vi "Vision Processing.vi"(4 "error in":errorcluster, 7 "Image Size":T6=enum."320x240") -> ()   [LabVIEW 2015]
doc: "This VI runs in parallel to other tasks. It gets images from the camera, processes them for color or shape and use that information to affect robot behavior."
uses:
  <vilib>/Rock Robotics/WPI/Camera/WPI_CameraImageSize.ctl
  Program Files (x86)/National Instruments/LabVIEW 2015/examples/FRC/roboRIO/Vision/2016 Vision Example/Vision Support Code/Camera Types.ctl
  <vilib>/Rock Robotics/WPI/Camera/WPI_CameraFrameRate.ctl
  Robot Global Data.vi
  <vilib>/vision/NI_Vision_Development_Module.lvlib
panel:
  out "Targets Angles":dbl[](array[numeric])
  in  "LED Color":T1={"Hue"={23.67058792990901, 48.923317529462665}, "Sat"={66.78571428571429, 255.0}, "Val"={48.571428571428584, 255.0}} {"Hue" scale=0.0..255.0 scale format="%#_3g"}
  out "Qualified Particles":i32
  in  "Score Threshold":dbl=75.0
  in  "Aspect Fudge Factor":dbl=1.0
  in  "Min Score Threshold":i32=75
  in  "Camera Type":T2=enum."MS HD3000 square"
  in  "Emphasize Limit Tests":bool=TRUE
  out "Masked":T3(plugin-control)
  out "Original Image":T3(plugin-control)
  in  "Display Images":bool
  out "Sorted Particle Scores":T4(array[cluster]) {"Moment Factor" format="%#_3g"; "Aspect Ratio" format="%#_3g"; "Area to CH" format="%#_3g"; "X" format="%#_3g"; "Y" format="%#_3g"}
  out "Highest Avg Score":dbl
  out "Detected Targets":T5(array[cluster]) {"Normalized Rect"."Numeric 5" format="%#_2g"; "Normalized Rect"."Numeric 3" format="%#_2g"; "Normalized Rect"."Numeric 2" format="%#_2g"; "Normalized Rect"."Numeric" format="%#_2g"}
  # "Density Profile"
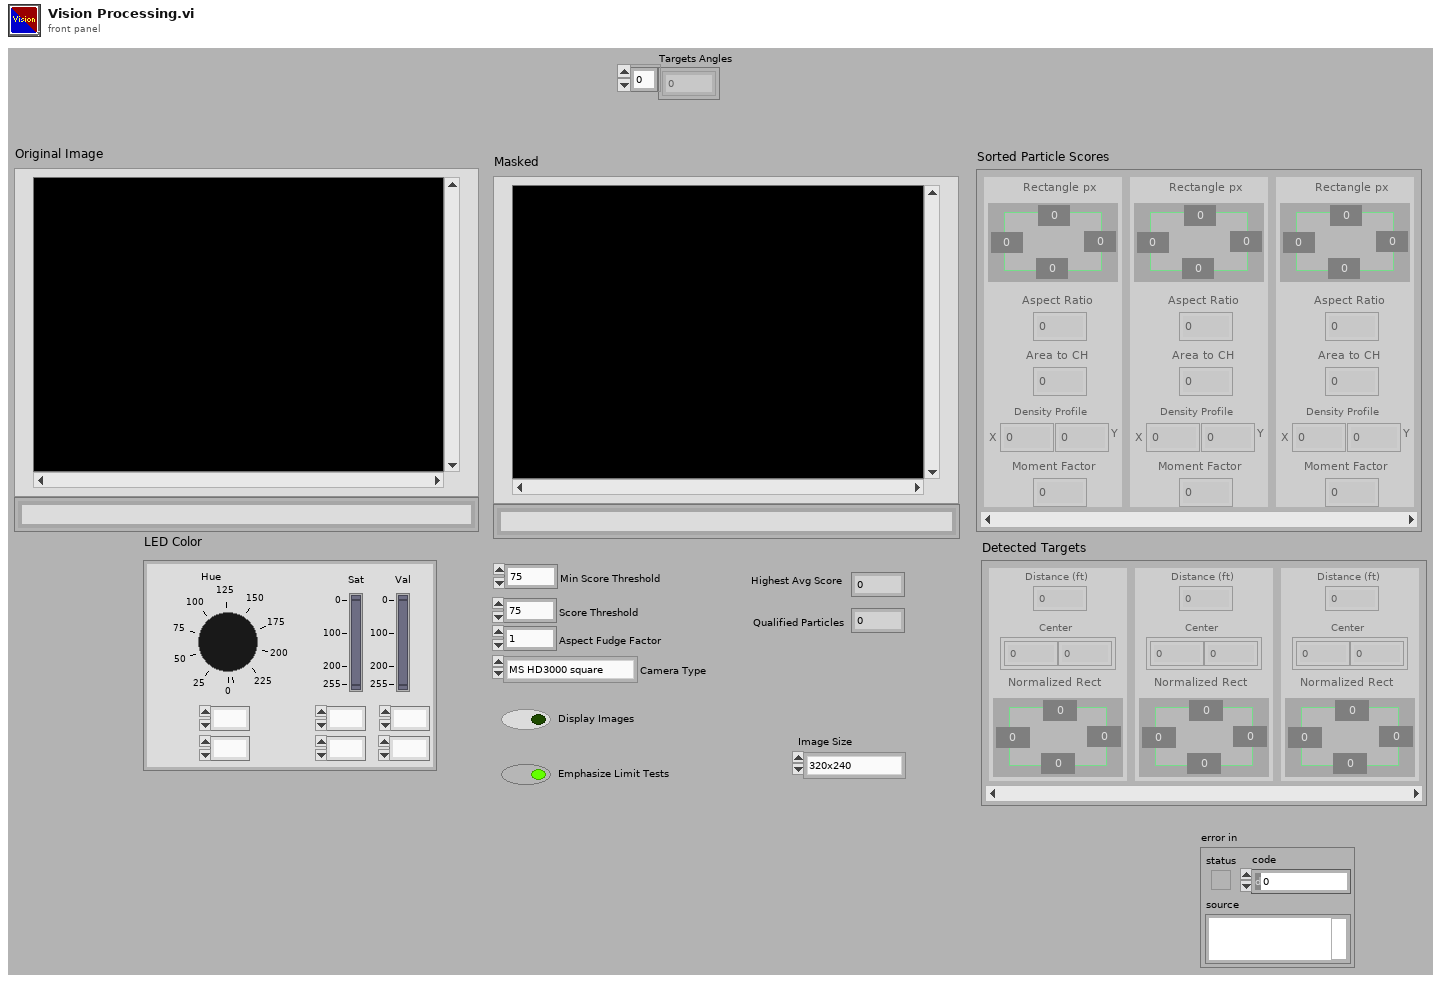
[diagram p1: front panel]
types:
  T1 = cluster{"Hue":cluster{dbl, dbl}, "Sat":cluster{dbl, dbl}, "Val":cluster{dbl, dbl}}
  T2 = typedef "Camera Types.ctl" = enum16{"206", "1011", "1013", "MS HD3000 square", "MS HD3000 640x480"}
  T3 = typedef "IMAQ Image.ctl" = refnum<image>
  T4 = cluster{"Rectangle px":cluster{"Numeric":dbl, "Numeric 2":dbl, "Numeric 3":dbl, "Numeric 5":dbl}, "Aspect Ratio":dbl, "Area to CH":dbl, "X":dbl, "Y":dbl, "Moment Factor":dbl}[]
  T5 = cluster{"Distance (ft)":dbl, "Center":cluster{dbl, dbl}, "Normalized Rect":cluster{"Numeric":dbl, "Numeric 2":dbl, "Numeric 3":dbl, "Numeric 5":dbl}}[]
  T6 = typedef "WPI_CameraImageSize.ctl" = enum16{"640x480", "320x240", "160x120", "Custom"}
  T7 = typedef "Particle Parameters" = i32
  T8 = typedef "Image Type" = u32
  T9 = typedef "WPI_CameraFrameRate.ctl" = u32
  T10 = typedef "WPI_CameraDevRef.ctl" = cluster{"Camera Address":string, "CameraStatus":errorcluster}
  T11 = cluster{"Bounding box":cluster{"left":dbl, "top":dbl, "right":dbl, "bottom":dbl}, "Aspect Ratio":dbl, "Area to CH":dbl, "X Mask":dbl, "Y Mask":dbl, "Moment":dbl}[]
  T12 = cluster{"Rectangle":cluster{"Numeric":dbl, "Numeric 2":dbl, "Numeric 3":dbl, "Numeric 5":dbl}, "L":dbl, "Area to CH":dbl, "X":dbl, "Y":dbl, "Moment Factor":dbl}[]
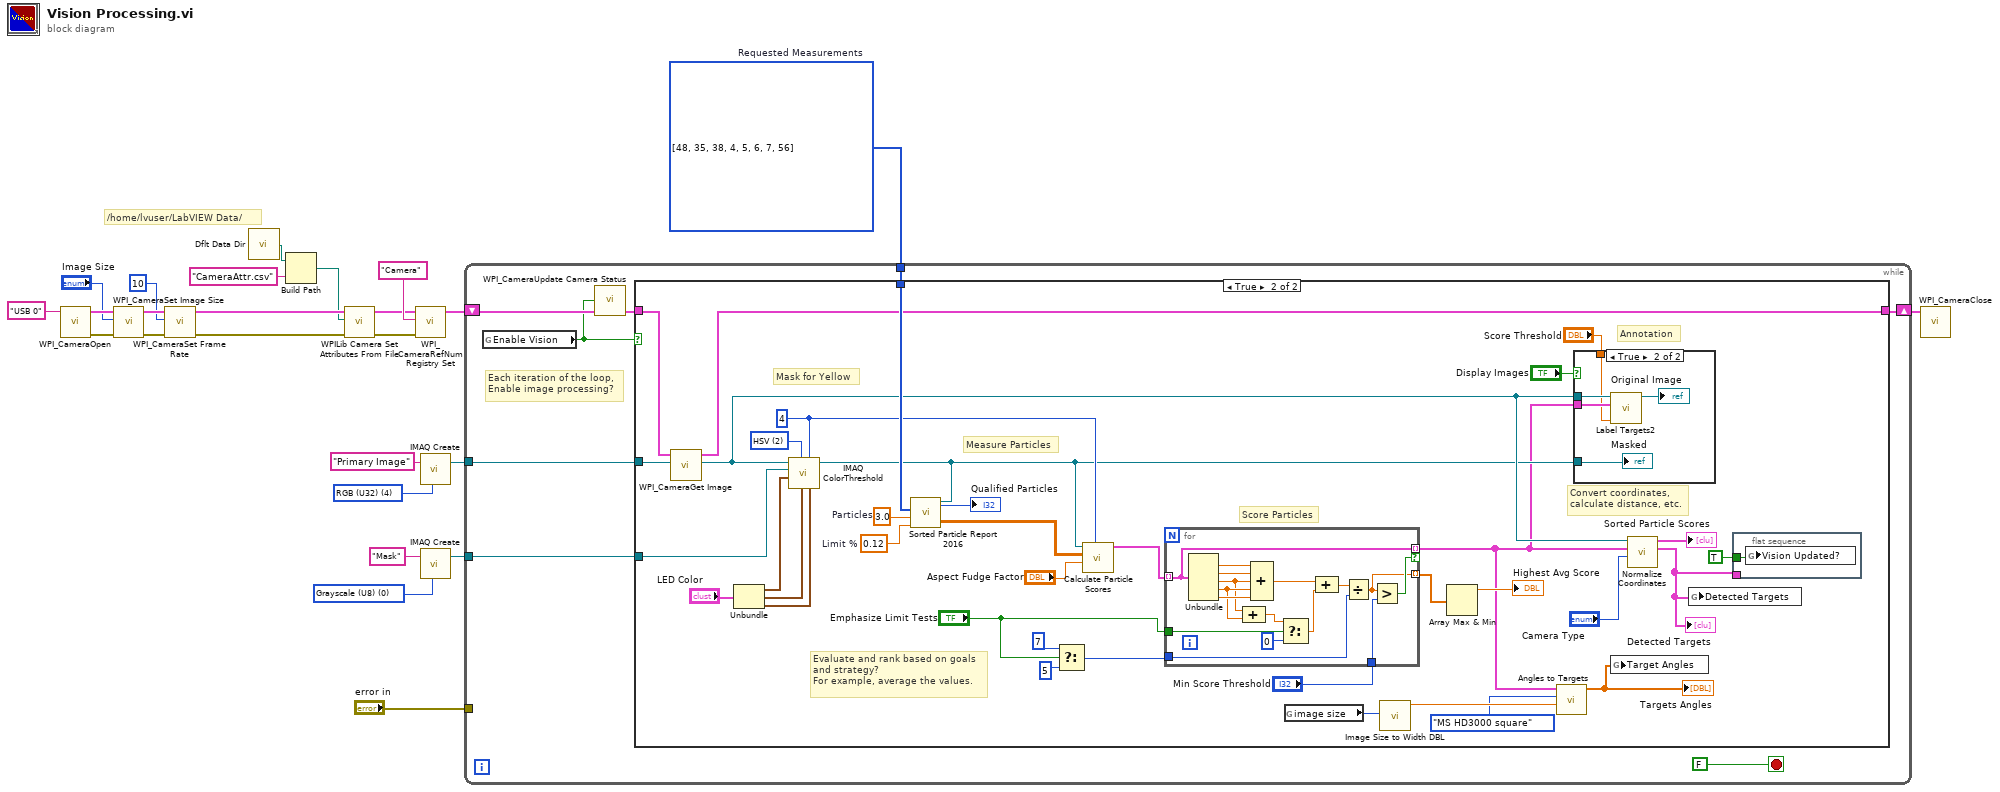
[diagram p0: block diagram]
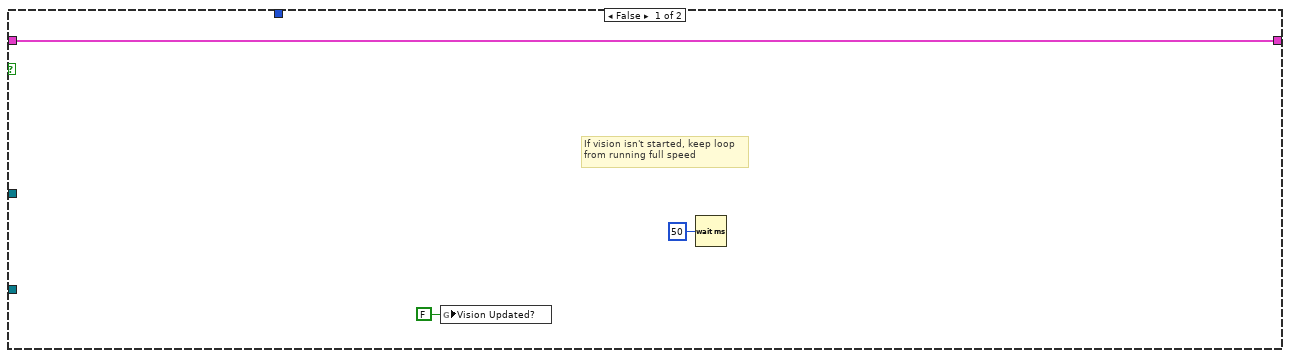
[diagram p2: hidden frame]
diagram:
  w1 = T7[] [48, 35, 38, 4, 5, 6, 7, 56] items=["Center of Mass X", "Center of Mass Y", "First Pixel X", "First Pixel Y", "Bounding Rect Left", "Bounding Rect Top", "Bounding Rect Right", "Bounding Rect Bottom", "Max Feret Diameter Start X", "Max Feret Diameter Start Y", "Max Feret Diameter End X", "Max Feret Diameter End Y", "Max Horiz. Segment Length Left", "Max Horiz. Segment Length Right", "Max Horiz. Segment Length Row", "-", "Bounding Rect Width", "Bounding Rect Height", "Bounding Rect Diagonal", "Perimeter", "Convex Hull Perimeter", "Holes' Perimeter", "Max Feret Diameter", "Equivalent Ellipse Major Axis", "Equivalent Ellipse Minor Axis", "Equivalent Ellipse Minor Axis (Feret)", "Equivalent Rect Long Side", "Equivalent Rect Short Side", "Equivalent Rect Diagonal", "Equivalent Rect Short Side (Feret)", "Average Horiz. Segment Length", "Average Vert. Segment Length", "Hydraulic Radius", "Waddel Disk Diameter", "-", "Area", "Holes' Area", "Particle & Holes' Area", "Convex Hull Area", "Image Area", "-", "Number of Holes", "Number of Horiz. Segments", "Number of Vert. Segments", "-", "Orientation", "Max Feret Diameter Orientation", "-", "% Area/Image Area", "% Area/(Particle & Holes' Area)", "Ratio of Equivalent Ellipse Axes", "Ratio of Equivalent Rect Sides", "-", "Elongation Factor", "Compactness Factor", "Heywood Circularity Factor", "Type Factor", "-", "Sum X", "Sum Y", "Sum XX", "Sum XY", "Sum YY", "Sum XXX", "Sum XXY", "Sum XYY", "Sum YYY", "-", "Moment of Inertia XX", "Moment of Inertia XY", "Moment of Inertia YY", "Moment of Inertia XXX", "Moment of Inertia XXY", "Moment of Inertia XYY", "Moment of Inertia YYY", "Norm. Moment of Inertia XX", "Norm. Moment of Inertia XY", "Norm. Moment of Inertia YY", "Norm. Moment of Inertia XXX", "Norm. Moment of Inertia XXY", "Norm. Moment of Inertia XYY", "Norm. Moment of Inertia YYY", "Hu Moment 1", "Hu Moment 2", "Hu Moment 3", "Hu Moment 4", "Hu Moment 5", "Hu Moment 6", "Hu Moment 7"]  # Requested Measurements
  w4 = T8 0 items=["Grayscale (U8)", "Grayscale (I16)", "Grayscale (SGL)", "Complex (CSG)", "RGB (U32)", "HSL (U32)", "RGB (U64)", "Grayscale (U16)"] ("Image Type")
  w25 = T8 4 items=["Grayscale (U8)", "Grayscale (I16)", "Grayscale (SGL)", "Complex (CSG)", "RGB (U32)", "HSL (U32)", "RGB (U64)"] ("Image Type")
  # "/home/lvuser/LabVIEW Data/"
  n1 = call <vilib>:"WPI_CameraOpen.vi"("Camera Address"="USB 0" ("format string")) -> ("error out"=w19:errorcluster, "CameraDevRef"=w20:T10)  [unwired: 1 in, 8 out]
  n2 = call <vilib>:"WPI_CameraSet Image Size.vi"("error in (no error)"=w19, "Image Size"="Image Size", "CameraDevRef"=w20) -> ("error out"=w18:errorcluster, "CameraDevRef Out"=w21:T10)  [unwired: 1 in, 6 out]
  n3 = call <vilib>:"WPI_CameraSet Frame Rate.vi"("error in (no error)"=w18, "Frame Rate (fps)"=T9 10, "CameraDevRef"=w21) -> ("error out"=w11:errorcluster, "CameraDevRef Out"=w12:T10)  [unwired: 7 out]
  n4 = call <vilib>:"Dflt Data Dir.vi"() -> ("App:Default Data Directory"=w8:path)
  n5 = Build Path(base path=w8, name or relative path="CameraAttr.csv") -> (appended path=w7:path)
  n6 = call "WPILib Camera Set Attributes From File.vi"("error in"=w11, "Config Path"=w7, "CameraDevRef"=w12) -> ("error out"=w9:errorcluster, "CameraDevRef"=w10:T10)  [unwired: 7 in]
  n7 = call <vilib>:"WPI_CameraRefNum Registry Set.vi"("error in (no error)"=w9, "refnum name"="Camera", "CameraDevRef"=w10) -> ("CameraDevRef"=w16:T10)  [unwired: 1 in, 7 out]
  n8 = call "IMAQ Create"("Image Name"="Primary Image", "Image Type"=w25) -> ("New Image"=w23:T3)  [unwired: 2 in, 2 out]
  n9 = call "IMAQ Create"("Image Name"="Mask", "Image Type"=w4) -> ("New Image"=w2:T3)  [unwired: 2 in, 2 out]
  n10 = while {
    shift-right: [w28] -> w5
    shift-left: w16 -> [w32]
    tunnel: w23 -> [w31]
    tunnel: "error in" -> [_]
    tunnel: w2 -> [w27]
    tunnel: w1 -> [w26]
    stop <- FALSE stop-if-true
    # "Each iteration of the loop,\nEnable image processing?"
    n11 = global read "Robot Global Data.vi" "Enable Vision"() -> (w29:bool)
    n12 = call <vilib>:"WPI_CameraUpdate Camera Status.vi"("CameraDevRef In"=w32, "Enable Vision"=w29) -> ("CameraDevRef Out"=w30:T10)  [unwired: 3 in]
    n13 = case shown="True" w29 {
      tunnel: w27 -> [_ w73]
      tunnel: w26 -> [_ w68]
      tunnel: w30 -> [w35 w64]
      tunnel: w31 -> [_ w63]
      tunnel: [w35 w62] -> w28
      frame False {
        # "If vision isn't started, keep loop\nfrom running full speed"
        n14 = global write "Robot Global Data.vi" "Vision Updated?"(FALSE ("Vision Updated?")) -> ()
        n15 = Wait (ms)(milliseconds to wait=u32 50) -> ()  [unwired: 1 out]
      }
      frame True {
        w48 = 4 ("Replace Value")
        w60 = u16 2 items=["RGB", "HSL", "HSV", "HSI"] ("Color Mode")
        w65 = 0.12  # Limit %
        w67 = 3.0  # Particles
        # "Evaluate and rank based on goals\nand strategy?\nFor example, average the values."
        # "Measure Particles"
        # "Convert coordinates,\ncalculate distance, etc."
        # "Annotation"
        # "Score Particles"
        # "Mask for Yellow"
        n16 = call <vilib>:"WPI_CameraGet Image.vi"("Image"=w63, "CameraDevRef"=w64) -> ("Image Out"=w50:T3, "CameraDevRef Out"=w62:T10)  [unwired: 7 in, 1 out]
        n17 = Unbundle("LED Color") -> ("Hue"=w72:cluster{dbl, dbl}, "Sat"=w71:cluster{dbl, dbl}, "Val"=w70:cluster{dbl, dbl})
        n18 = call "IMAQ ColorThreshold"("Blue or Luma or Val or Inten Range"=w70, "Replace Value"=w48, "Green or Sat Range"=w71, "Color Mode"=w60, "Red or Hue Range"=w72, "Image Dst"=w73, "Image Src"=w50) -> ("Image Dst Out"=w46:T3)  [unwired: 3 in, 1 out]
        n19 = call "Sorted Particle Report 2016.vi"("Min Area Size %"=w65, "Particle Count Limit"=w67, "Pixel Measurements"=w68, "Image in"=w46) -> ("Sorted Data"=w59:dbl[][], "Particles"=→"Qualified Particles":i32)
        n20 = Select(t=7, s="Emphasize Limit Tests", f=5) -> (s? t:f=w54:i32)
        n21 = call "Calculate Particle Scores.vi"("Pixel Value"=w48, "Aspect Fudge Factor"="Aspect Fudge Factor", "Sorted Data"=w59, "Image in"=w46) -> ("Scores"=w57:T11)  [unwired: 7 in]
        n22 = for {
          tunnel: w57 -> [w88] mode=indexing
          tunnel: [w88] -> w43 mode=indexing if=w87
          tunnel: [w86] -> w44 mode=indexing
          tunnel: w54 -> [w85]
          tunnel: "Min Score Threshold" -> [w84]
          tunnel: "Emphasize Limit Tests" -> [w77]
          n23 = Unbundle(w88) -> ("Aspect Ratio"=w90:dbl, "Area to CH"=w89:dbl, "X Mask"=w79:dbl, "Y Mask"=w80:dbl, "Moment"=w81:dbl)  [unwired: 1 out]
          n24 = Compound Arithmetic op=ADD(w79, w80) -> (w78:dbl)
          n25 = Compound Arithmetic op=ADD(w90, w89, w79, w80, w81) -> (w83:dbl)
          n26 = Select(t=w78, s=w77, f=0) -> (s? t:f=w76:dbl)
          n27 = Compound Arithmetic op=ADD(w83, w76) -> (w82:dbl)
          n28 = Divide(x=w82, y=w85) -> (x/y=w86:dbl)
          n29 = Greater?(x=w86, y=w84) -> (0:w87:bool)
        }
        n30 = global read "Robot Global Data.vi" "image size"() -> (w42:T6)
        n31 = call "Image Size to Width DBL.vi"("image size"=w42) -> ("Numeric"=w41:dbl)  [unwired: 10 in]
        n32 = Array Max & Min(array=w44) -> (max value=→"Highest Avg Score":dbl)  [unwired: 3 out]
        n33 = call "Angles to Targets.vi"("Pixel Width"=w41, "Camera Type"=Camera_Types."MS HD3000 square", "Targets In"=w43) -> ("Target Angle"=w39:dbl[])  [unwired: 8 in]
        "Targets Angles" <- w39
        n34 = case shown="True" "Display Images" {
          tunnel: w50 -> [_ w95]
          tunnel: w43 -> [_ w93]
          tunnel: "Score Threshold" -> [_ w92]
          tunnel: w46 -> [_ w91]
          frame False {
          }
          frame True {
            n35 = call "Label Targets2.vi"("Score Threshold"=w92, "Targets"=w93, "Image in"=w95) -> ("Image out"=→"Original Image":T3)  [unwired: 8 in]
            "Masked" <- w91
          }
        }
        n36 = global write "Robot Global Data.vi" "Target Angles"(w39) -> ()
        n37 = call "Normalize Coordinates.vi"("Camera Type"="Camera Type", "Targets"=w43, "Image in"=w50) -> ("Found Targets"=w38:T5, "Sorted Scores"=→"Sorted Particle Scores":T12)  [unwired: 7 in]
        "Detected Targets" <- w38
        n38 = global write "Robot Global Data.vi" "Detected Targets"(w38) -> ()
        n39 = flat-sequence {
          tunnel: w38 -> [_]
          tunnel: TRUE -> [w74]
          frame #0 {
            n40 = global write "Robot Global Data.vi" "Vision Updated?"(w74) -> ()
          }
        }
      }
    }
  }
  n41 = call <vilib>:"WPI_CameraClose.vi"("CameraDevRef"=w5) -> ()  [unwired: 1 in, 10 out]
